vi "Do Action.vi"(8 "error in (no error)":errorcluster, 10 "Action Configuration":cluster{"Action":T1, "Configuration":variant}, 11 "Main Display in":refnum<class "Main Display.lvclass">) -> (0 "error out":errorcluster, 3 "Main Display out":refnum<class "Main Display.lvclass">)   [LabVIEW 2016, in "Assert API Components.lvlib" / "Assert Display.lvlib" / "Main Display.lvlib" / "Main Display.lvclass"]
uses:
  Main Display.lvclass
  Actions.ctl
  Main Display.lvclass/Main Display.ctl
  Timing Engine/Timing Engine Messages/Timer Update Msg/Timer Update Msg.lvclass/Timer Update Msg.ctl
  <vilib>/ActorFramework/Message Enqueuer/Message Enqueuer.lvclass/Message Enqueuer.ctl
  <vilib>/ActorFramework/Message Enqueuer/Enqueue.vi
  Timing Engine/Timing Engine Messages/Timer Update Msg/Timer Update Msg.lvclass
  C:/Program Files (x86)/National Instruments/LabVIEW 2016/vi.lib/ActorFramework/Message/Message.lvclass
  <vilib>/ActorFramework/Message Priority Queue/Priority Enqueue.vi
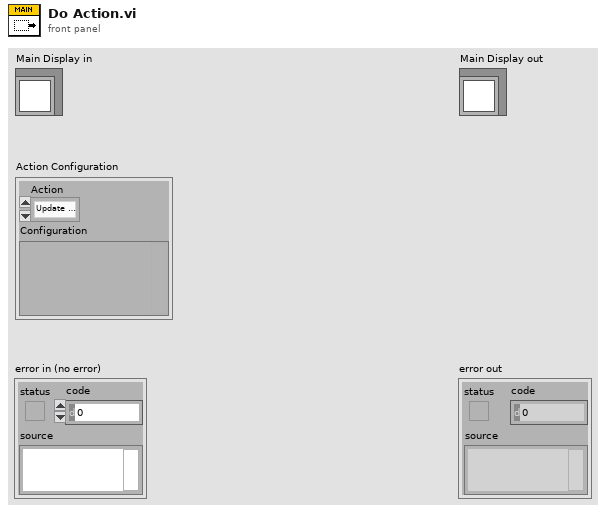
[diagram p1: front panel]
types:
  T1 = typedef "Assert API Components.lvlib/Assert Display.lvlib/Main Display.lvlib/Main Display.lvclass/Actions.ctl" = enum16{"Update Timeout"}
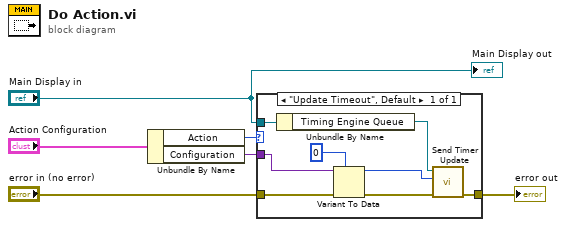
[diagram p0: block diagram]
diagram:
  n1 = Unbundle By Name("Action Configuration") -> ("Action"=w5:T1, "Configuration"=w4:variant)
  n2 = case shown="\"Update Timeout\", Default" w5 {
    tunnel: w4 -> [w14]
    tunnel: "error in (no error)" -> [w12]
    tunnel: "Main Display in" -> [w11]
    tunnel: [w7] -> w1
    frame "Update Timeout", Default {
      n3 = Unbundle By Name(w11) -> ("Timing Engine Queue"=w10:refnum<class "Message Enqueuer.lvclass">)
      n4 = Variant To Data(error in=w12, type=0, Variant=w14) -> (data=w9:i32, error out=w8:errorcluster)
      n5 = call "Send Timer Update.vi"("error in (no error)"=w8, "Timeout Value"=w9, "Message Enqueuer"=w10) -> ("error out"=w7:errorcluster)  [unwired: 7 in, 1 out]
    }
  }
  "error out" <- w1
  "Main Display out" <- "Main Display in"
